vi "check data size.vi"(11 "data type":T1) -> (3 "bytes":i32)   [LabVIEW 2013, in "EthernetIP Channel.lvclass"]
uses:
  EthernetIP Channel.lvclass
  <vilib>/NI/Tag Bus/tag/Data Type.ctl
  <vilib>/NI/Tag Bus/tag/tag descriptor.lvclass
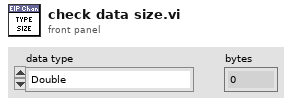
[diagram p1: front panel]
types:
  T1 = typedef "tag bus.lvlib/tag descriptor.lvclass/Data Type.ctl" = enum16{"Double", "Single", "I64", "I32", "I16", "I8", "U64", "U32", "U16", "U8", "Boolean", "String", "Array of Double", "Array of Single", "Array of I64", "Array of I32", "Array of I16", "Array of I8", "Array of U64", "Array of U32", "Array of U16", "Array of U8", "Array of Boolean", "Array of String"}
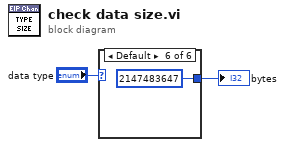
[diagram p0: block diagram]
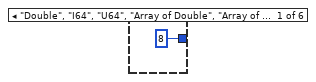
[diagram p2: hidden frame]
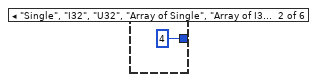
[diagram p3: hidden frame]
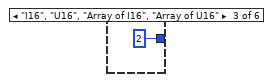
[diagram p4: hidden frame]
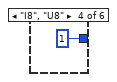
[diagram p5: hidden frame]
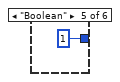
[diagram p6: hidden frame]
diagram:
  n1 = case shown="Default" "data type" {
    tunnel: [8 ("x") 4 ("x") 2 ("x") 1 ("x") 1 ("x") 2147483647 ("x")] -> w2
    frame "Double", "I64", "U64", "Array of Double", "Array of I64", "Array of U64" {
    }
    frame "Single", "I32", "U32", "Array of Single", "Array of I32", "Array of U32" {
    }
    frame "I16", "U16", "Array of I16", "Array of U16" {
    }
    frame "I8", "U8" {
    }
    frame "Boolean" {
    }
    frame Default {
    }
  }
  "bytes" <- w2
